vi "get system info.vi"(8 "error in":errorcluster) -> (0 "error out":errorcluster, 3 "System Info":T1)   [LabVIEW 2013]
uses:
  <vilib>/NI/TagWebClient/API/JSON Formats/System Info Results.ctl
  <vilib>/Analysis/baseanly.llb/Mean (DBL).vi
  <vilib>/nisyscfg/Find Hardware.vi
  <vilib>/Analysis/NI_AALBase.lvlib
  <vilib>/nisyscfg/nisyscfg.lvlib
  <resource>/objmgr/motionsysapi.rc
  <vilib>/NI/TagWebClient/API/tagweb client API.lvlib
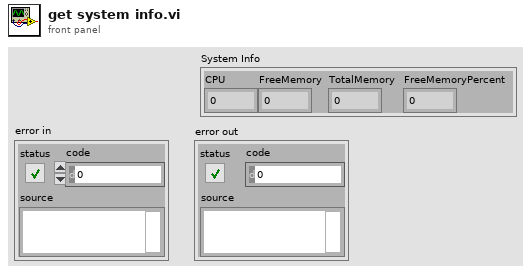
[diagram p1: front panel]
types:
  T1 = typedef "tagweb client API.lvlib/System Info Results.ctl" = cluster{"CPU":dbl, "FreeMemory":dbl, "TotalMemory":dbl, "FreeMemoryPercent":dbl}
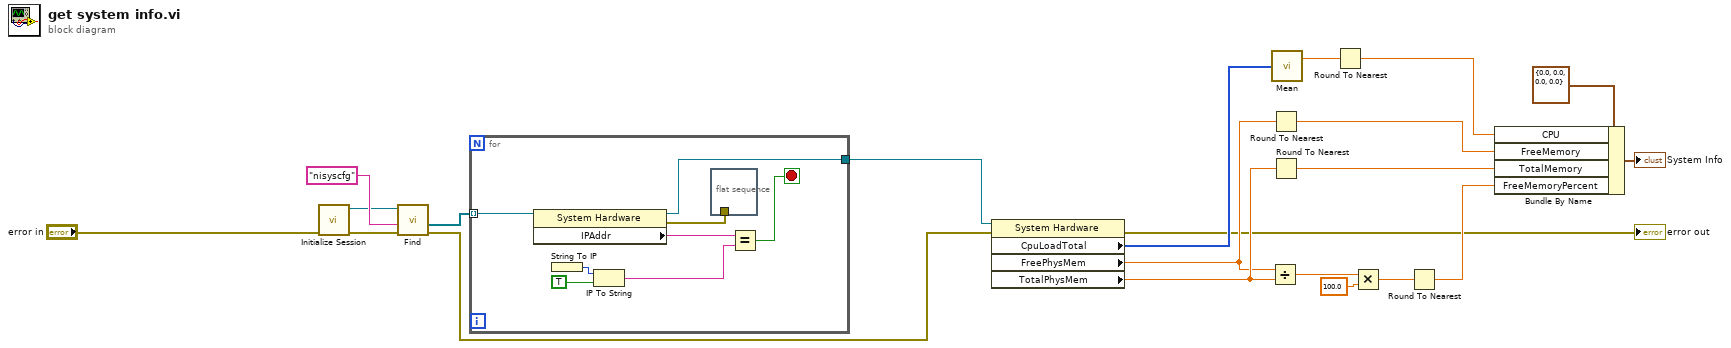
[diagram p0: block diagram]
diagram:
  n1 = call <vilib>:"Initialize Session.vi"("error in (no error)"="error in") -> ("error out"=w1:errorcluster, "Session out"=w2:refnum<k21>)  [unwired: 9 in]
  n2 = call-poly <vilib>:"Find.vi"("error in (no error)"=w1, "Experts"="nisyscfg" ("experts"), "Session in"=w2) -> ("error out"=w21:errorcluster, "Resources out"=w4:refnum<k20>[])  [unwired: 5 in, 2 out]
  n3 = for {
    tunnel: w4 -> [w29] mode=indexing
    tunnel: [w24] -> w20
    stop <- w23 stop-if-true
    n4 = property class="System Hardware"(reference=w29) -> (reference out=w24:refnum<k20>, error out=w22:errorcluster, "IPAddr"=w26:string)  [unwired: 1 in]
    n5 = String To IP() -> (0:w27:u32)  [unwired: 1 in]
    n6 = IP To String(1:TRUE ("dot notation? (F)"), 2:w27) -> (0:w25:string)
    n7 = flat-sequence {
      tunnel: w22 -> [_]
      frame #0 {
      }
    }
    n8 = Equal?(x=w26, y=w25) -> (x = y?=w23:bool)
  }
  n9 = property class="System Hardware"(reference=w20, error in=w21) -> (error out=→"error out":errorcluster, "CpuLoadTotal"=w13:u32[], "FreePhysMem"=w15:dbl, "TotalPhysMem"=w16:dbl)  [unwired: 1 out]
  n10 = Divide(x=w15, y=w16) -> (x/y=w17:dbl)
  n11 = Round To Nearest(number=w15) -> (nearest integer value=w9:dbl)
  n12 = Round To Nearest(number=w16) -> (nearest integer value=w10:dbl)
  n13 = call-poly <vilib>:"Mean.vi"("X"=w13) -> ("mean"=w14:dbl)  [unwired: 1 out]
  n14 = Round To Nearest(number=w14) -> (nearest integer value=w12:dbl)
  n15 = Multiply(x=w17, y=100.0) -> (x*y=w19:dbl)
  n16 = Round To Nearest(number=w19) -> (nearest integer value=w11:dbl)
  n17 = Bundle By Name(cluster=T1 {"CPU"=0.0, "FreeMemory"=0.0, "TotalMemory"=0.0, "FreeMemoryPercent"=0.0} ("System Info"), "CPU"=w12, "FreeMemory"=w9, "TotalMemory"=w10, "FreeMemoryPercent"=w11) -> (→"System Info":T1)
